vi "Set Scalar Configuration.vi"(8 "error in (no error)":errorcluster, 9 "index":i32, 10 "transfer configuration":T1={"name"="Transfer"}, 11 "Core Transfers Configuration in":refnum<class "Core Transfers Configuration.lvclass">) -> (0 "error out":errorcluster, 3 "Core Transfers Configuration out":refnum<class "Core Transfers Configuration.lvclass">)   [LabVIEW 2017, in "DSF Core.lvlib" / "Core Transfers Configuration.lvclass"]
uses:
  Core Transfers Configuration.lvclass
  Configuration.ctl
  Core Transfers Configuration.lvclass/Core Transfers Configuration.ctl
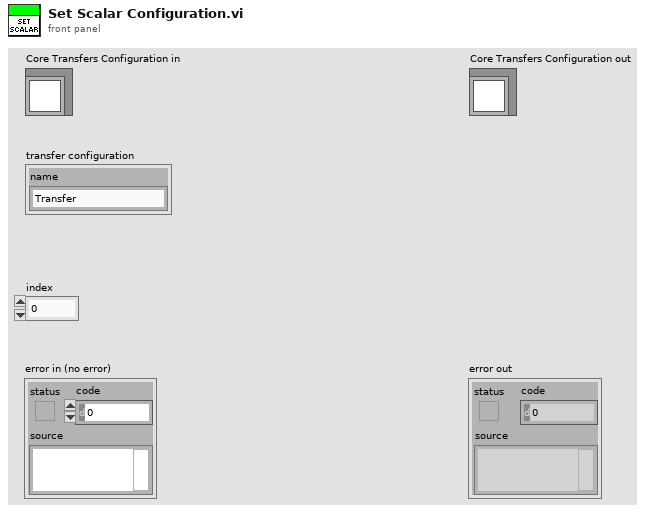
[diagram p1: front panel]
types:
  T1 = typedef "DSF Core.lvlib/Core Transfers Configuration.lvclass/Configuration.ctl" = cluster{"name":string}
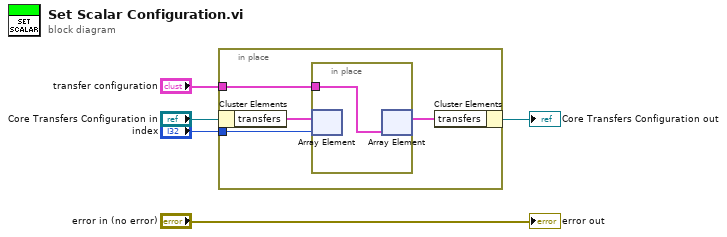
[diagram p0: block diagram]
diagram:
  n1 = in-place {
    in-place-border: "index" -> [w8]
    in-place-border: "transfer configuration" -> [w7]
    n2 = in-place-cluster #1("Core Transfers Configuration in") -> ("transfers"=w9:T1[])
    n3 = in-place {
      in-place-border: w7 -> [w10]
      n4 = in-place-array #2(w9, w8) -> ()  [unwired: 1 out]
      n5 = in-place-array #2(w10) -> (w6:T1[])  [unwired: 1 out]
    }
    n6 = in-place-cluster #1("transfers"=w6) -> (→"Core Transfers Configuration out":refnum<class "Core Transfers Configuration.lvclass">)
  }
  "error out" <- "error in (no error)"
